vi "Add Control Caption.vi"(8 "error in (no error)":errorcluster, 11 "Listbox in":refnum<class "Listbox.lvclass">) -> (0 "error out":errorcluster, 3 "Listbox out":refnum<class "Listbox.lvclass">)   [LabVIEW 2017, in "Localization.lvlib" / "Listbox.lvclass"]
doc: "VI for override that is supposed to do go throgh and create the Caption for the specific VI. Then the caption is set as visible and the label is hidden.\n\nChoose Movement Consulting, LLC"
uses:
  Listbox.lvclass
  C:/Apps/CMC/OpenSource/Localization/Control Info/Control Info.lvclass
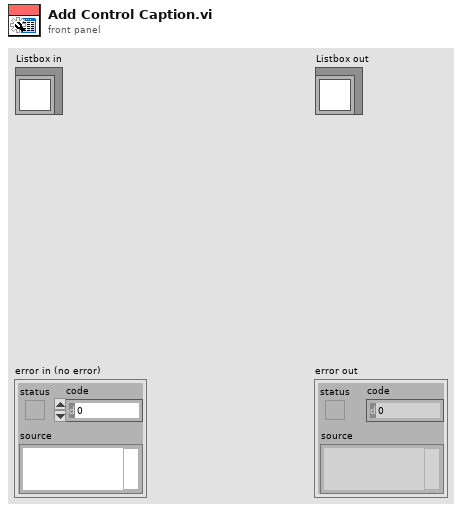
[diagram p1: front panel]
types:
  T1 = typedef "LVPositionTypeDef.ctl" = cluster{"Left":i32, "Top":i32}
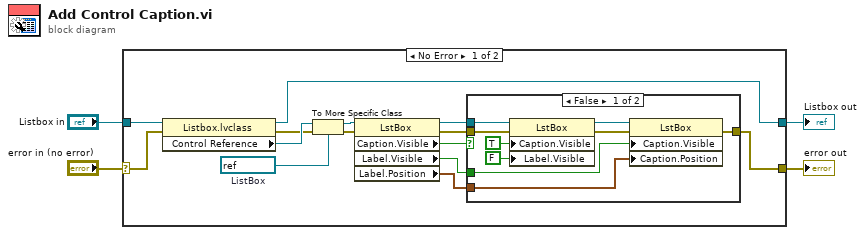
[diagram p0: block diagram]
diagram:
  n1 = case shown="No Error" "error in (no error)" {
    selector: "error in (no error)" -> [w13 w30]
    tunnel: "Listbox in" -> [w12 w29]
    tunnel: [w9 w29] -> w2
    tunnel: [w7 w30] -> w1
    frame No Error {
      w14 = refnum<vi> refnum  # ListBox
      n2 = property class="Listbox.lvclass"(reference=w12, error in=w13) -> (reference out=w9:refnum<class "Listbox.lvclass">, error out=w17:errorcluster, "Control Reference"=w18:refnum<vi>)
      n3 = To More Specific Class(target class=w14, reference=w18, error in=w17) -> (specific class reference=w15:refnum<vi>, error out=w16:errorcluster)
      n4 = property class="LstBox"(reference=w15, error in=w16) -> (reference out=w8:refnum<vi>, error out=w10:errorcluster, "Caption.Visible"=w11:bool, "Label.Visible"=w6:bool, "Label.Position"=w5:T1)
      n5 = case shown="False" w11 {
        tunnel: w10 -> [w26 w28]
        tunnel: w8 -> [w27 _]
        tunnel: [w23 w28] -> w7
        tunnel: w6 -> [w20 _]
        tunnel: w5 -> [w19 _]
        frame False {
          n6 = property class="LstBox"(reference=w27, error in=w26, "Caption.Visible"=TRUE, "Label.Visible"=FALSE) -> (reference out=w22:refnum<vi>, error out=w21:errorcluster)
          n7 = property class="LstBox"(reference=w22, error in=w21, "Caption.Visible"=w20, "Caption.Position"=w19) -> (error out=w23:errorcluster)  [unwired: 1 out]
        }
        frame True {
        }
      }
    }
    frame Error {
    }
  }
  "error out" <- w1
  "Listbox out" <- w2
